vi "RT Driver VI_Test.vi"(7 "Operation":T1, 11 "Device Reference in":T2 format="%.0x") -> (0 "Error Code":i32)   [LabVIEW 2013, in "OPC UA Client Engine.lvlib"]
uses:
  OPC UA Client Engine.lvlib
  <vilib>/NI Veristand/Custom Device API/Custom Device Item Ref.ctl
  <vilib>/NI Veristand/Custom Device API/Hardware Interface Driver VI Operation.ctl
  <vilib>/OPCUA/NI OPC UA Client.lvlib
  <vilib>/NI VeriStand/Custom Device Tools/Custom Device Utility Library/Custom Device Utility Library.lvlib
  <vilib>/NI Veristand/Custom Device API/Custom Device API.lvlib
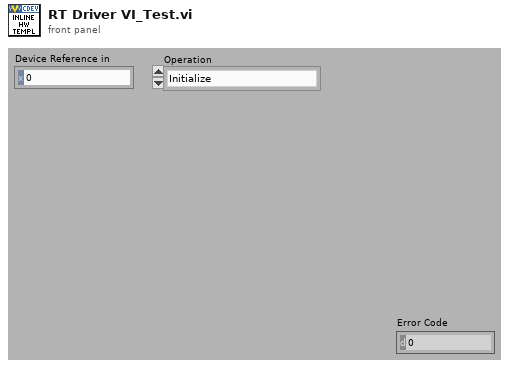
[diagram p1: front panel]
types:
  T1 = typedef "Custom Device API.lvlib/Hardware Interface Driver VI Operation.ctl" = enum16{"Initialize", "Start", "Read Data from HW", "Write Data to HW", "Close"}
  T2 = typedef "Custom Device API.lvlib/Custom Device Item Ref.ctl" = u64
  T3 = cluster{"message mode":enum16{"None", "Sign", "Sign and Encrypt"}, "security":enum16{"Basic256", "Basic128Rsa15"}}
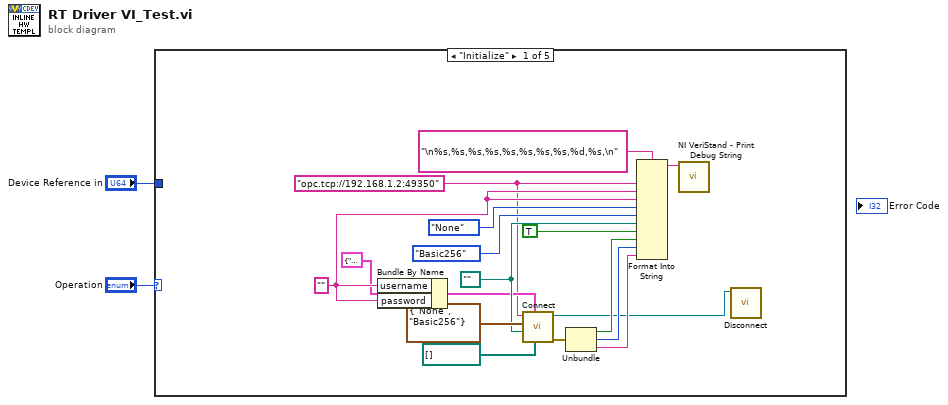
[diagram p0: block diagram]
diagram:
  n1 = case shown="\"Initialize\"" "Operation" {
    tunnel: "Device Reference in" -> [_ _ _ _ _]
    frame "Initialize" {
      w3 = "opc.tcp://192.168.1.2:49350" ("concatenated string")
      w14 = "" ("Connection.Properties.Password")
      w11 = path "" ("client certificate file")
      n2 = Bundle By Name(cluster=cluster{"username":string, "password":string} {"username"="", "password"=""} ("username/password"), "username"=w14, "password"=w14) -> (w6:cluster{"username":string, "password":string})
      n3 = call <vilib>:"Connect.vi"("trusted server certificates"=path[] [], "username/password"=w6, "client certificate file"=w11, "security policy"=T3 {"message mode"=enum."None", "security"=enum."Basic256"}, "server endpoint URL"=w3) -> ("error out"=w16:errorcluster, "OPC UA client refnum out"=w4:refnum<k21>)  [unwired: 4 in, 1 out]
      n4 = Unbundle(w16) -> ("status"=w17:bool, "code"=w18:i32, "source"=w19:string)
      n5 = Format Into String(format string="\n%s,%s,%s,%s,%s,%s,%s,%s,%d,%s,\n", w3, w14, w14, enum16{"None", "Sign", "Sign and Encrypt"}."None" ("Connection.Properties.Message Mode"), enum16{"Basic256", "Basic128Rsa15"}."Basic256" ("Connection.Properties.Security"), w11, TRUE ("input 7"), w17, w18, w19) -> (resulting string=w8:string)  [unwired: 2 in, 1 out]
      n6 = call <vilib>:"NI VeriStand - Print Debug String.vi"("Message"=w8) -> ()  [unwired: 10 in, 1 out]
      n7 = call <vilib>:"Disconnect.vi"("OPC UA client refnum in"=w4) -> ()  [unwired: 10 in, 1 out]
    }
    frame "Start" {
    }
    frame "Read Data from HW" {
    }
    frame "Write Data to HW" {
    }
    frame "Close" {
    }
  }
